vi "01-SimpleStateMachine.vi"() -> ()   [LabVIEW 2017]
uses:
  Support/01-Typedef.ctl
panel:
  in  "stop":bool
  in  "Msg Button":bool
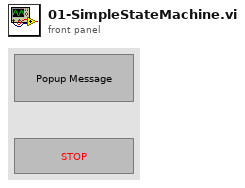
[diagram p1: front panel]
types:
  T1 = typedef "01-Typedef.ctl" = enum16{"Init", "Button", "Idle", "Exit"}
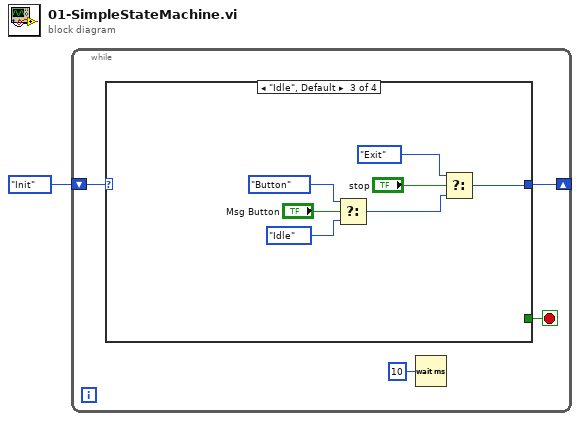
[diagram p0: block diagram]
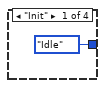
[diagram p2: hidden frame]
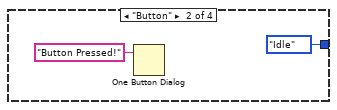
[diagram p3: hidden frame]
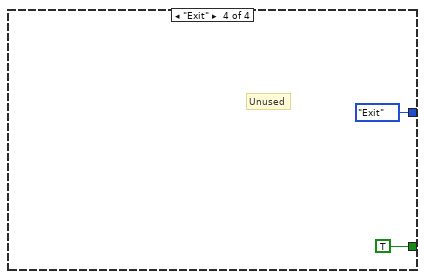
[diagram p4: hidden frame]
diagram:
  n1 = while {
    shift-right: [w2] -> _
    shift-left: 01-Typedef."Init" ("Enum") -> [w5]
    stop <- w4 stop-if-true
    n2 = case shown="\"Idle\", Default" w5 {
      tunnel: [_ _ _ TRUE] -> w4
      tunnel: [01-Typedef."Idle" ("Enum") 01-Typedef."Idle" ("Enum") w11 01-Typedef."Exit" ("Enum")] -> w2
      frame "Init" {
      }
      frame "Button" {
        n3 = One Button Dialog(message="Button Pressed!") -> ()  [unwired: 1 in, 1 out]
      }
      frame "Idle", Default {
        n4 = Select(t=01-Typedef."Button" ("Enum"), s="Msg Button", f=01-Typedef."Idle" ("Enum")) -> (s? t:f=w14:T1)
        n5 = Select(t=01-Typedef."Exit", s="stop", f=w14) -> (s? t:f=w11:T1)
      }
      frame "Exit" {
        # "Unused"
      }
    }
    n6 = Wait (ms)(milliseconds to wait=u32 10) -> ()  [unwired: 1 out]
  }
